vi "Read Measurement.vi"   [LabVIEW 2010, in "Agilent 3458.lvlib"]
doc: "Reads one or more measurements from the DMM."
uses:
  <instrlib>/Agilent 3458/Agilent 3458.lvlib
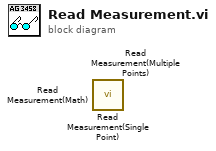
[diagram p0: block diagram]
diagram:
  n1 = call <instrlib>:"Read Measurement(Single Point).vi"() -> ()  [unwired: 13 in, 3 out]
  n2 = call <instrlib>:"Read Measurement(Multiple Points).vi"() -> ()  [unwired: 13 in, 3 out]
  n3 = call <instrlib>:"Read Measurement(Math).vi"() -> ()  [unwired: 9 in, 7 out]
